vi "ModbusRxDataFIFO.vi"   [LabVIEW 2016]
uses:
  <vilib>/rvi/Emulation/niFpgaGetClockAttributes.vi
  <vilib>/rvi/Emulation/niFpgaSctlEmulationGetInTimedLoop.vi
  <vilib>/rvi/Emulation/niFpgaEmulationReportErrorSimple.vi
  <vilib>/rvi/Emulation/niFpgaCriticalErrorInLSC.vi
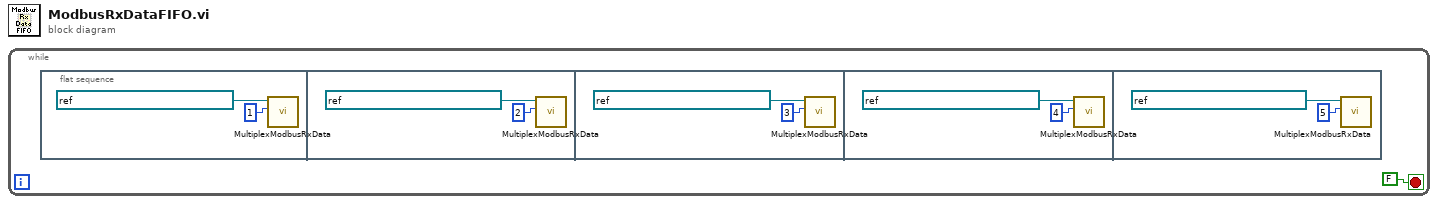
[diagram p0: block diagram]
diagram:
  n1 = while {
    stop <- FALSE stop-if-true
    n2 = flat-sequence {
      frame #0 {
        n3 = call "MultiplexModbusRxData.vi"("ID"=u16 1, "InputFIFO"=refnum<k21> "ModbusSubnetARxDataFIFO") -> ()  [unwired: 10 in]
      }
      frame #1 {
        n4 = call "MultiplexModbusRxData.vi"("ID"=u16 2, "InputFIFO"=refnum<k21> "ModbusSubnetBRxDataFIFO") -> ()  [unwired: 10 in]
      }
      frame #2 {
        n5 = call "MultiplexModbusRxData.vi"("ID"=u16 3, "InputFIFO"=refnum<k21> "ModbusSubnetCRxDataFIFO") -> ()  [unwired: 10 in]
      }
      frame #3 {
        n6 = call "MultiplexModbusRxData.vi"("ID"=u16 4, "InputFIFO"=refnum<k21> "ModbusSubnetDRxDataFIFO") -> ()  [unwired: 10 in]
      }
      frame #4 {
        n7 = call "MultiplexModbusRxData.vi"("ID"=u16 5, "InputFIFO"=refnum<k21> "ModbusSubnetERxDataFIFO") -> ()  [unwired: 10 in]
      }
    }
  }
